vi "CommunicationTool-Ver1.vi"(0 "VISA资源名称":refnum<visa-resource-name>="COM29", 1 "SN":string, 2 "ModelNumber":string, 5 "通信协议名称":string, 9 "DelayTime":u32=1000, 11 "error in":errorcluster, 12 "Debug":bool) -> (3 "字符串数值":bool, 4 "响应":string="ÿÿÿÿÿÿÿÿÿÿÿÿÿÿÿÿÿÿÿÿÿÿÿÿÿÿÿ", 6 "反馈结果":bool, 10 "CMD":string, 14 "data":string, 15 "error out":errorcluster)   [LabVIEW 2013]
doc: "本范例根据用户指示，对串口执行读写操作。范例运行时可按下“写入”或“读取”按钮，以及修改“读数”。\n\n设置的串口参数必须匹配连接仪器或设备的参数。本范例中，“读数”参数可指定串口读取的字节数。如端口字节超过指定的字节数，超出部分将不会被读取。如端口字节数少于指定的字节数，将返回超时错误。\n\n本范例可扩展流控制选项以包括XON和XOFF，从而允许用户选择控制字符。同时，用户可启用或禁用中止符。部分设备需要通过终止符确定命令字符串的结束位置。部分设备将发送终止符以说明待读取数据的末端。本范例演示了缓冲区中检测到终止符时，结束“读取”操作或添加终止符至“写入”数据末端的方法。"
uses:
  <vilib>/Utility/NIReport.llb/NI_report.lvclass
  Ctl/Paractl.ctl
  GlobValue.vi
  <vilib>/Utility/error.llb/Error Cluster From Error Code.vi
  <vilib>/addons/_office/excel.llb/Excel Get Data ([str]).vi
  <vilib>/ErrorRing/Error Ring.xnode
  <vilib>/addons/_office/NI_ReportGenerationToolkit.lvlib
  <vilib>/Utility/NIReport.llb/Excel/NI_Excel.lvclass
panel:
  out "字符串 2":string
  out "日期/时间字符串":string
  out "times":dbl
  out "反馈前段":string
  out "Time(ms)":u32
  out "SerNO":string
  out "硬件版本":string
  out "CCID":string="PASS"
  out "生产日期":string
  out "字符串":string
  out "x-y":u32
  out "读取缓冲区":string
  in  "命令列表":u16(ring)=17 items=["启动自动化测试", "退出自动化测试", "进入待机模式", "进入工作模式", "查询ACC IO状态", "GPS定位查询", "查询GPS定位时间", "GPS可见星数", "上网模块自检", "上网模块信号强度", "查询上网模块GPRS状态", "WIFI模块自检", "外部Flash测试", "查询电池电压", "查询电源电压", "CHARGE_CTL置低", "CHARGE_CTL置高", "查询CHARGE_WAKE状态", "3G_PWR_CTL输出低电平", "3G_PWR_CTL输出高电平", "3G_RST输出低电平", "3G_RST输出高电平", "查询ANT1_S状态", "查询ANT0_S状态", "GPS_PWREN输出低电平", "GPS_PWREN输出高电平", "CAN通信接收", "CAN通信发送", "重启", "U_CTL输出低电平", "U_CTL输出高电平", "OBD_CTL输出低电平", "OBD_CTL输出高电平", "OBD_STB输出低电平", "OBD_STB输出高电平", "3G_EN输出低电平", "3G_EN输出高电平", "写入主机条码", "读出主机条码", "写入生产日期", "读出生产日期", "读出CCID", "写入终端ID", "读出终端ID", "写入硬件版本", "读出硬件版本", "查看TBC文件", "进入休眠模式", "写入APN1", "写入APN2", "读出APN1", "读出APN2", "写入WIFI名称", "写入WIFI密码", "WIFI模块自检", "读出WIFI名称", "读出WIFI密码", "查询4G固件版本", "查询平台登录状态", "读OPEN软件版本", "写入车辆TUID", "读出车辆TUID", "查询MCU软件版本", "写入证书编号", "读出证书编号", "写入供应商代码", "读出供应商代码", "写入零部件号", "读出零部件号", "读出WIFI MAC地址", "OPEN模块自检", "切断备电供电", "恢复备电供电", "检测备电电压", "检测B+电源电压", "查询平台登录状态", "SRS碰撞检测", "启动测试回环Speak", "启动测试回环Aux", "关闭测试回环", "E-call状态返回", "MIC_CTL输出低电平", "MIC_CTL输出高电平", "读取IMSI号"]
  out "Write":bool
  out "Read":bool
  out "ConfigPath":string="C:\\Users\\dell\\Desktop\\ExcelReport.vi"
  out "命令":string
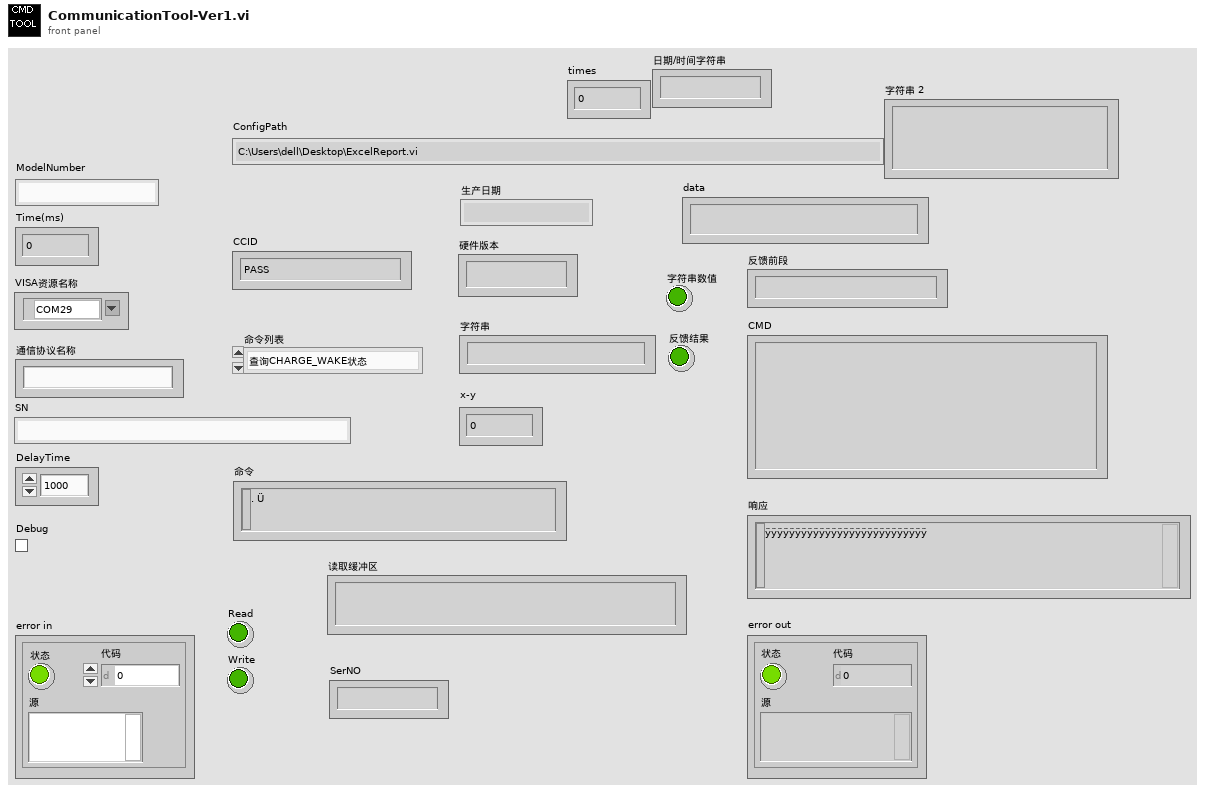
[diagram p1: front panel]
types:
  T1 = enum32{"invalid app kind", "Development System", "Run Time System", "Student Edition", "Embedded LabVIEW", "Evaluation", "Custom"}
  T2 = enum16{"maximized", "minimized", "normal", "no change"}
  T3 = enum16{"Standard Report", "HTML", "Word", "Excel"}
  T4 = typedef "Paractl.ctl" = enum16{"Fw Ver", "HW Ver", "CCID", "WiFiName", "DevID", "SN", "TUID", "CertifID", "PdTime", "Provider", "WiFiPassword", "Imei", "AuthCode", "Reserved1", "Reserved2", "Reserved3"}
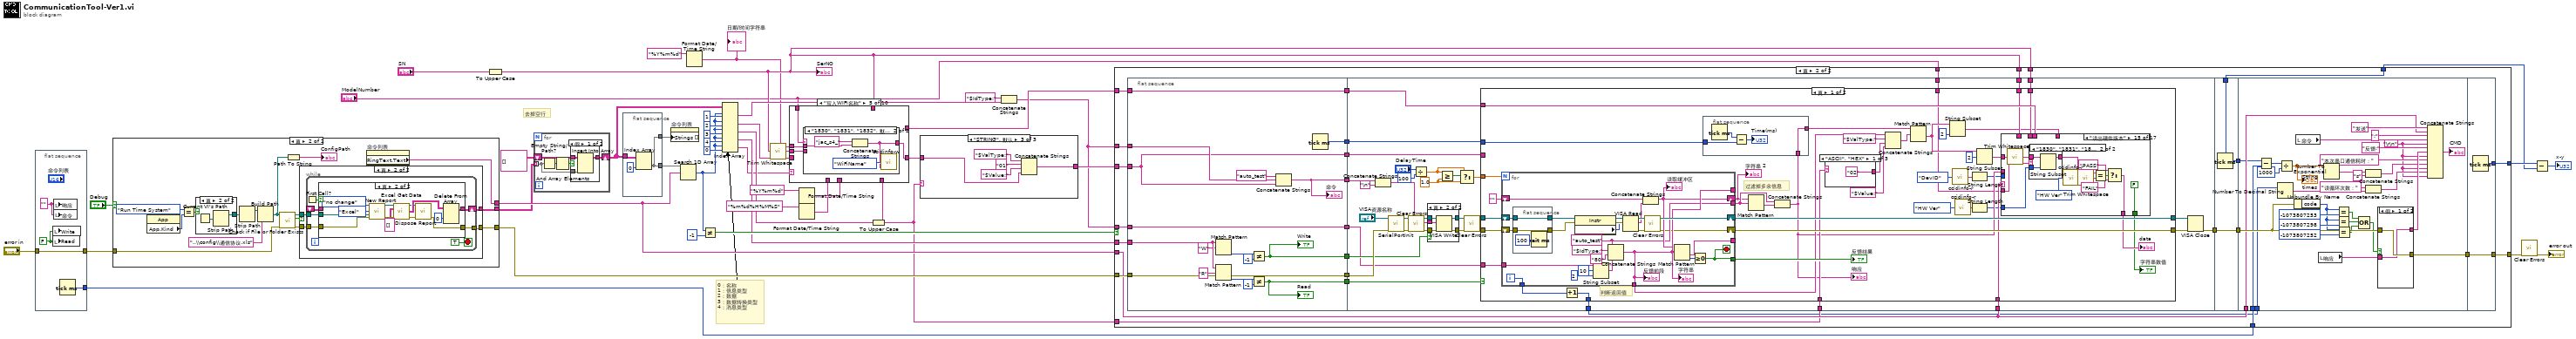
[diagram p0: block diagram]
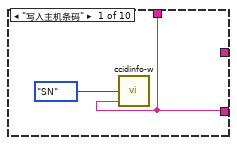
[diagram p2: hidden frame]
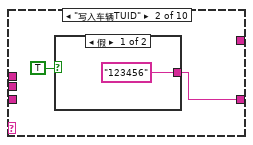
[diagram p3: hidden frame]
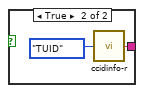
[diagram p4: hidden frame]
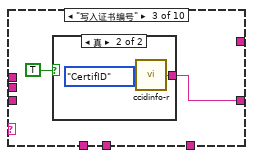
[diagram p5: hidden frame]
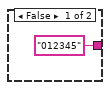
[diagram p6: hidden frame]
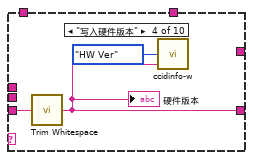
[diagram p7: hidden frame]
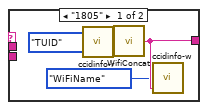
[diagram p8: hidden frame]
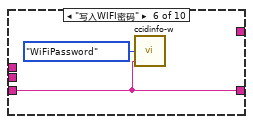
[diagram p9: hidden frame]
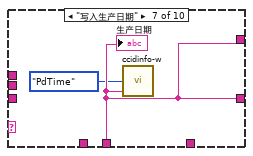
[diagram p10: hidden frame]
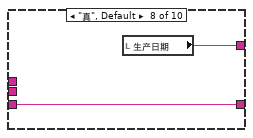
[diagram p11: hidden frame]
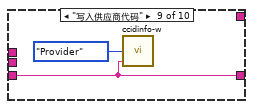
[diagram p12: hidden frame]
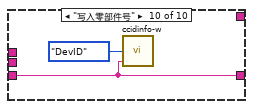
[diagram p13: hidden frame]
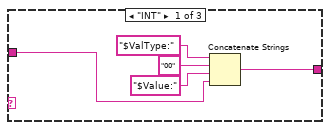
[diagram p15: hidden frame]
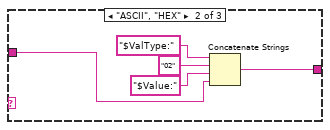
[diagram p16: hidden frame]
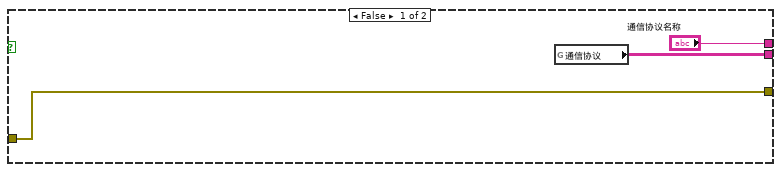
[diagram p17: hidden frame]
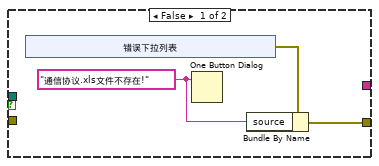
[diagram p18: hidden frame]
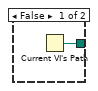
[diagram p20: hidden frame]
diagram:
  # "0：名称\n1：信息类型\n2：数据\n3：数据转换类型\n4：消息类型"
  # "去掉空行"
  n1 = flat-sequence {
    tunnel: "error in" -> [w47]
    tunnel: [w47] -> w43
    tunnel: [w46] -> w5
    frame #0 {
      w49 = FALSE ("Read")
      w48 = "" ("响应")
      n2 = local write "Write"(w49) -> ()
      n3 = local write "Read"(w49) -> ()
      n4 = local write "响应"(w48) -> ()
      n5 = local write "命令"(w48) -> ()
      n6 = Tick Count (ms)() -> (millisecond timer value=w46:u32)
    }
  }
  n7 = case shown="真" "Debug" {
    tunnel: [w51 w56] -> w41
    tunnel: w43 -> [w51 w55]
    tunnel: ["通信协议名称" w53] -> w34
    tunnel: [w50 w54] -> w19
    frame False {
      n8 = global read "GlobValue.vi" "通信协议"() -> (w50:string[][])
    }
    frame True {
      n9 = property class="App"() -> ("App.Kind"=w65:T1)  [unwired: 2 in, 2 out]
      n10 = Equal?(x=T1."Run Time System" ("y"), y=w65) -> (x = y?=w67:bool)
      n11 = case shown="真" w67 {
        tunnel: [w101 w103] -> w66
        frame False {
          n12 = Current VI's Path() -> (path=w101:path)
        }
        frame True {
          n13 = Current VI's Path() -> (path=w102:path)
          n14 = Strip Path(path=w102) -> (stripped path=w103:path)  [unwired: 1 out]
        }
      }
      n15 = Strip Path(path=w66) -> (stripped path=w60:path)  [unwired: 1 out]
      n16 = Build Path(base path=w60, name or relative path="..\\config\\通信协议.xls" ("连接的字符串")) -> (appended path=w62:path)
      n17 = call <vilib>:"Check if File or Folder Exists.vi"("error in (no error)"=w55, "path"=w62) -> ("error out"=w57:errorcluster, "file or folder exists?"=w59:bool, "dup path"=w58:path)  [unwired: 7 out]
      n18 = Path To String(path=w62) -> (string=→"ConfigPath":string)
      n19 = case shown="真" w59 {
        tunnel: w58 -> [_ w78]
        tunnel: w57 -> [_ w77]
        tunnel: [w69 w76] -> w56
        tunnel: [_ w75] -> w54
        frame False {
          w70 = "通信协议.xls文件不存在!" ("消息")
          n20 = xnode "错误下拉列表"() -> ("错误输出"=w68:errorcluster)
          n21 = One Button Dialog(message=w70) -> ()  [unwired: 1 in, 1 out]
          n22 = Bundle By Name(cluster=w68, "source"=w70) -> (w69:errorcluster)
        }
        frame True {
          n23 = while {
            tunnel: w78 -> [w84]
            tunnel: [w83] -> w76
            tunnel: w77 -> [w82]
            shift-right: [w85] -> w75
            shift-left: _ -> [w80]
            stop <- TRUE stop-if-true
            n24 = First Call?() -> (First Call?: T/F=w79:bool)
            n25 = case shown="真" w79 {
              tunnel: [w87 w91] -> w85
              tunnel: w84 -> [_ w90]
              tunnel: [w86 w89] -> w83
              tunnel: w82 -> [w86 w88]
              tunnel: w80 -> [w87 _]
              frame False {
              }
              frame True {
                n26 = call <vilib>:"New Report.vi"("window state (normal)"=T2."no change", "report type"=T3."Excel", "template (empty)"=w90, "error in (no error)"=w88) -> ("report out"=w96:refnum<class "NI_report.lvclass">, "error out"=w97:errorcluster)  [unwired: 2 in, 8 out]
                n27 = call-poly <vilib>:"Excel Get Data.vi"("report in"=w96, "data type"=string[][] [], "error in (no error)"=w97) -> ("report out"=w93:refnum<class "NI_report.lvclass">, "data"=w98:string[][], "error out"=w92:errorcluster)  [unwired: 10 in]
                n28 = call-dynamic "Dispose Report.vi"("report in"=w93, "error in (no error)"=w92) -> ("error out"=w89:errorcluster)  [unwired: 3 in, 10 out]
                n29 = Delete From Array(array=w98, index (row)=0 ("索引 (行)")) -> (array with subset deleted=w91:string[][])  [unwired: 2 in, 1 out]
              }
            }
          }
        }
      }
      n30 = property on="命令列表" class="Ring (严格)"() -> ("RingText.Text"=w53:string)  [unwired: 2 in, 2 out]
    }
  }
  n31 = To Upper Case(1:"SN") -> (0:w11:string)
  "SerNO" <- w11
  n32 = for {
    tunnel: w19 -> [w104] mode=indexing
    shift-right: [w107] -> w27
    shift-left: string[][] [] -> [w108]
    n33 = Empty String/Path?(string/path=w104) -> (empty?=w106:bool[])
    n34 = And Array Elements(Boolean array=w106) -> (logical AND=w105:bool)
    n35 = case shown="假" w105 {
      tunnel: w108 -> [w111 w112]
      tunnel: [w110 w112] -> w107
      tunnel: w104 -> [w109 _]
      frame False {
        n36 = Insert Into Array(array=w111, new element=w109) -> (w110:string[][])  [unwired: 2 in]
      }
      frame True {
      }
    }
  }
  n37 = flat-sequence {
    tunnel: [w113] -> w33
    tunnel: w27 -> [w114]
    tunnel: [w113] -> w17
    frame #0 {
      n38 = Index Array(array=w114, index (col)=0 ("禁用的索引 (列)")) -> (element=w113:string[])  [unwired: 1 in]
    }
  }
  n39 = property on="命令列表" class="Ring (严格)"("Strings []"=w17) -> ()  [unwired: 2 in, 2 out]
  n40 = Search 1D Array(1D array=w33, element=w34) -> (index of element=w16:i32)  [unwired: 1 in]
  n41 = Format Date/Time String(time format string (%c)="%Y%m%d" ("时间格式字符串(%c)")) -> (date/time string=w1:string)  [unwired: 2 in]
  "日期/时间字符串" <- w1
  n42 = Not Equal?(x=w16, y=-1) -> (x != y?=w36:bool)
  n43 = Index Array(array=w27, index (row) #1=w16, index (col) #1=1 ("索引 (列)"), index (row) #2=w16, index (col) #2=2 ("索引 (列)"), index (row) #3=w16, index (col) #3=3 ("索引 (列)"), index (row) #4=w16, index (col) #4=4 ("禁用的索引 (列)"), index (row) #5=w16, index (col) #5=0 ("禁用的索引 (列)")) -> (element #1=w13:string, element #2=w23:string, element #3=w29:string, element #4=w31:string, element #5=w15:string)
  n44 = call <vilib>:"Trim Whitespace.vi"("string"=w11) -> ("trimmed string"=w3:string)  [unwired: 1 in]
  n45 = Format Date/Time String(time format string (%c)="%Y%m%d" ("时间格式字符串(%c)")) -> (date/time string=w9:string)  [unwired: 2 in]
  n46 = Format Date/Time String(time format string (%c)="%m%d%H%M%S" ("时间格式字符串(%c)")) -> (date/time string=w7:string)  [unwired: 2 in]
  n47 = To Upper Case(1:w29) -> (0:w18:string)
  n48 = case shown="\"写入WIFI名称\"" w15 {
    tunnel: w23 -> [_ _ _ w130 _ w144 _ w148 w150 w152]
    tunnel: [w117 w119 w124 w129 w134 w144 w146 w148 w150 w152] -> w20
    tunnel: [_ _ _ _ _ _ w146 w147 _ _] -> w21
    tunnel: w11 -> [w117 _ _ _ _ _ _ _ _ _]
    tunnel: w3 -> [_ _ _ _ w132 _ _ _ _ _]
    tunnel: w18 -> [_ _ _ _ _ _ _ _ _ _]
    tunnel: w9 -> [_ _ _ _ _ _ w146 _ _ _]
    tunnel: "ModelNumber" -> [_ _ _ _ w133 _ _ _ _ _]
    tunnel: w7 -> [_ _ _ _ _ _ _ _ _ _]
    tunnel: w1 -> [_ _ _ _ w131 _ _ _ _ _]
    frame "写入主机条码" {
      n49 = call "ccidinfo-w.vi"("Data"=w117, "Data Type"=Paractl."SN") -> ()  [unwired: 2 in]
    }
    frame "写入车辆TUID" {
      n50 = case shown="假" TRUE {
        tunnel: ["123456" ("Data") w122] -> w119
        frame False {
        }
        frame True {
          n51 = call "ccidinfo-r.vi"("Data Type"=Paractl."TUID") -> ("Data"=w122:string)
        }
      }
    }
    frame "写入证书编号" {
      n52 = case shown="真" TRUE {
        tunnel: ["012345" ("Data") w127] -> w124
        frame False {
        }
        frame True {
          n53 = call "ccidinfo-r.vi"("Data Type"=Paractl."CertifID") -> ("Data"=w127:string)
        }
      }
    }
    frame "写入硬件版本" {
      n54 = call <vilib>:"Trim Whitespace.vi"("string"=w130) -> ("trimmed string"=w129:string)  [unwired: 1 in]
      "硬件版本" <- w129
      n55 = call "ccidinfo-w.vi"("Data"=w129, "Data Type"=Paractl."HW Ver") -> ()  [unwired: 2 in]
    }
    frame "写入WIFI名称" {
      n56 = case shown="\"1830\", \"1831\", \"1832\", 默认" w133 {
        tunnel: [w137 w141] -> w134
        tunnel: w132 -> [_ _]
        tunnel: w131 -> [_ w139]
        frame "1805" {
          n57 = call "ccidinfo-r.vi"("Data Type"=Paractl."TUID") -> ("Data"=w138:string)
          n58 = call "WifiConcat.vi"("TUID"=w138) -> ("WIFIName"=w137:string)
          n59 = call "ccidinfo-w.vi"("Data"=w137, "Data Type"=Paractl."WiFiName") -> ()  [unwired: 2 in]
        }
        frame "1830", "1831", "1832", Default {
          n60 = Concatenate Strings("jac_s4_" ("SerNO 2"), w139) -> (w141:string)
          n61 = call "ccidinfo-w.vi"("Data"=w141, "Data Type"=Paractl."WiFiName") -> ()  [unwired: 2 in]
        }
      }
    }
    frame "写入WIFI密码" {
      n62 = call "ccidinfo-w.vi"("Data"=w144, "Data Type"=Paractl."WiFiPassword") -> ()  [unwired: 2 in]
    }
    frame "写入生产日期" {
      n63 = call "ccidinfo-w.vi"("Data"=w146, "Data Type"=Paractl."PdTime") -> ()  [unwired: 2 in]
      "生产日期" <- w146
    }
    frame "真", Default {
      n64 = local read "生产日期"() -> (w147:string)
    }
    frame "写入供应商代码" {
      n65 = call "ccidinfo-w.vi"("Data"=w150, "Data Type"=Paractl."Provider") -> ()  [unwired: 2 in]
    }
    frame "写入零部件号" {
      n66 = call "ccidinfo-w.vi"("Data"=w152, "Data Type"=Paractl."DevID") -> ()  [unwired: 2 in]
    }
  }
  n67 = case shown="\"STRING\", 默认" w18 {
    tunnel: [w153 w158 w163] -> w35
    tunnel: w20 -> [w154 w159 w164]
    frame "INT" {
      n68 = Concatenate Strings("$ValType:", "00", "$Value:", w154) -> (w153:string)
    }
    frame "ASCII", "HEX" {
      n69 = Concatenate Strings("$ValType:", "02", "$Value:", w159) -> (w158:string)
    }
    frame "STRING", Default {
      n70 = Concatenate Strings("$ValType:", "01", "$Value:", w164) -> (w163:string)
    }
  }
  n71 = Concatenate Strings("$IdType:", w13) -> (w12:string)
  n72 = case shown="真" w36 {
    tunnel: w34 -> [w172 w191]
    tunnel: w12 -> [_ w200]
    tunnel: w35 -> [_ w199]
    tunnel: w41 -> [_ w198]
    tunnel: [w168 w196] -> w45
    tunnel: w31 -> [_ w195]
    tunnel: w18 -> [_ w177]
    tunnel: [_ w187] -> w42
    tunnel: [_ w186] -> w26
    tunnel: w21 -> [_ w185]
    tunnel: w11 -> [_ w183]
    tunnel: w11 -> [_ w182]
    tunnel: w12 -> [_ w178]
    tunnel: "ModelNumber" -> [_ w176]
    tunnel: w5 -> [_ w174]
    frame False {
      (unwired) "FF" ("响应")
      n73 = Concatenate Strings(w172, "名称不存在" ("消息")) -> (w169:string)
      n74 = One Button Dialog(message=w169) -> ()  [unwired: 1 in, 1 out]
      n75 = Bundle By Name(cluster=errorcluster {"status"=TRUE, "code"=5000, "source"=""} ("error in 1 (no error)"), "source"=w169) -> (w168:errorcluster)
    }
    frame True {
      n76 = flat-sequence {
        tunnel: w200 -> [w206]
        tunnel: w199 -> [w204]
        tunnel: w198 -> [w217]
        tunnel: [w217] -> w197
        tunnel: w195 -> [w216]
        tunnel: [w209] -> w194
        tunnel: [w208] -> w193
        tunnel: [w207] -> w192
        tunnel: w185 -> [w205]
        tunnel: [w205] -> w184
        tunnel: [w204] -> w181
        tunnel: [w203] -> w180
        tunnel: [w201] -> w179
        tunnel: w178 -> [w201]
        tunnel: w197 -> [w247]
        tunnel: w194 -> [w242]
        tunnel: w193 -> [w245]
        tunnel: [w246] -> w190
        tunnel: w192 -> [w226]
        tunnel: w191 -> [w233]
        tunnel: w184 -> [w232]
        tunnel: w183 -> [w231]
        tunnel: w182 -> [w230]
        tunnel: w181 -> [w229]
        tunnel: w180 -> [w228]
        tunnel: w179 -> [w223]
        tunnel: w177 -> [w222]
        tunnel: w176 -> [w221]
        tunnel: [w220] -> w173
        tunnel: w190 -> [w486]
        tunnel: [w486] -> w189
        tunnel: [w485] -> w186
        tunnel: [w485] -> w175
        tunnel: w189 -> [w512]
        tunnel: w191 -> [w506]
        tunnel: [w513] -> w188
        tunnel: w175 -> [w500]
        tunnel: w174 -> [w499]
        tunnel: w173 -> [w492]
        tunnel: [w524] -> w196
        tunnel: w188 -> [w524]
        tunnel: [w523] -> w187
        frame #0 {
          n77 = Match Pattern(string=w216, regular expression="W" ("正则表达式")) -> (offset past match=w210:i32)  [unwired: 1 in, 3 out]
          n78 = Match Pattern(string=w216, regular expression="R" ("正则表达式")) -> (offset past match=w211:i32)  [unwired: 1 in, 3 out]
          n79 = Not Equal?(x=w210, y=-1) -> (x != y?=w209:bool)
          "Write" <- w209
          n80 = Not Equal?(x=w211, y=-1) -> (x != y?=w208:bool)
          "Read" <- w208
          n81 = Concatenate Strings("auto_test", w206, w204) -> (w207:string)
          "命令" <- w207
          n82 = Tick Count (ms)() -> (millisecond timer value=w203:u32)
        }
        frame #1 {
          w239 = 1.0 ("y")
          n83 = Concatenate Strings(w226, "\n") -> (w224:string)
          n84 = call "SerialPortInit.vi"("错误输入"=w247, "COMIn"="VISA资源名称") -> ("错误输出"=w243:errorcluster, "COMOut"=w244:refnum<visa-resource-name>)  [unwired: 8 in]
          n85 = call <vilib>:"Clear Errors.vi"("error in (no error)"=w243) -> ("error out"=w219:errorcluster)  [unwired: 6 in]
          n86 = Divide(x="DelayTime", y=u32 100) -> (x/y=w238:dbl)
          n87 = case shown="真" w242 {
            tunnel: w244 -> [w251 w256]
            tunnel: [w251 w255] -> w241
            tunnel: [w250 w254] -> w240
            tunnel: w219 -> [w250 w253]
            tunnel: w224 -> [_ w252]
            frame False {
            }
            frame True {
              n88 = VISA Write(VISA resource name=w256, write buffer=w252, error in (no error)=w253) -> (VISA resource name out=w255:refnum<visa-resource-name>, error out=w254:errorcluster)  [unwired: 1 out]
            }
          }
          n89 = Greater Or Equal?(x=w238, y=w239) -> (x >= y?=w237:bool)
          n90 = Select(t=w238, s=w237, f=w239) -> (s? t:f=w234:dbl)
          n91 = call <vilib>:"Clear Errors.vi"("error in (no error)"=w240) -> ("error out"=w218:errorcluster)  [unwired: 6 in]
          n92 = case shown="真" w245 {
            tunnel: [w295 w484] -> w248
            tunnel: w241 -> [w294 w484]
            tunnel: [w296 w483] -> w249
            tunnel: w218 -> [w293 w483]
            tunnel: w234 -> [w291 _]
            tunnel: w233 -> [w290 _]
            tunnel: w232 -> [w287 _]
            tunnel: w231 -> [w286 _]
            tunnel: w230 -> [w285 _]
            tunnel: w229 -> [_ _]
            tunnel: w228 -> [w284 _]
            tunnel: w223 -> [w281 _]
            tunnel: w222 -> [w280 _]
            tunnel: w221 -> [w266 _]
            tunnel: [w264 _] -> w220
            frame True {
              # "过滤掉多余信息"
              # "判断返回值"
              n93 = for {
                N: w291 -> [_]
                shift-right: [w455] -> w296
                shift-left: w293 -> [w470]
                shift-right: [w458] -> w257
                shift-left: "" ("read buffer") -> [w474]
                shift-right: [w478] -> w295
                shift-left: w294 -> [w469]
                tunnel: [w468] -> w282
                tunnel: [w459] -> _
                tunnel: w281 -> [w466]
                tunnel: [w460] -> _
                tunnel: [w459] -> w279
                tunnel: [w457] -> w269
                tunnel: [w456] -> w265
                i -> [w456]
                stop <- w468 stop-if-true
                w457 = "auto_test"
                n94 = flat-sequence {
                  tunnel: w470 -> [w482]
                  tunnel: [w482] -> w471
                  tunnel: [w481] -> w472
                  tunnel: w469 -> [w481]
                  frame #0 {
                    n95 = Wait (ms)(milliseconds to wait=u32 100 ("等待时间（毫秒）")) -> ()  [unwired: 1 out]
                  }
                }
                n96 = property class="Instr"(reference=w472, error in=w471) -> (reference out=w477:refnum<visa-resource-name>, error out=w476:errorcluster, "Serial Settings:Number of Bytes at Serial Port"=w475:u32)
                n97 = String Subset(string=w466, offset (0)=10 ("偏移量(0)"), length (rest)=2 ("长度（剩余）")) -> (substring=w467:string)
                n98 = Concatenate Strings(w457, "$IdType:", "80" ("字符串"), w467) -> (w459:string)
                "字符串" <- w459
                "反馈前段" <- w459
                n99 = VISA Read(VISA resource name=w477, byte count=w475, error in (no error)=w476) -> (VISA resource name out=w478:refnum<visa-resource-name>, read buffer=w473:string, error out=w479:errorcluster)  [unwired: 1 out]
                n100 = Concatenate Strings(w474, w473) -> (w458:string)
                "读取缓冲区" <- w458
                n101 = call <vilib>:"Clear Errors.vi"("error in (no error)"=w479) -> ("error out"=w455:errorcluster)  [unwired: 6 in]
                n102 = Match Pattern(string=w458, regular expression=w459) -> (after substring=w460:string, offset past match=w461:i32)  [unwired: 1 in, 2 out]
                n103 = Greater Or Equal To 0?(x=w461) -> (x >= 0?=w468:bool)
              }
              "反馈结果" <- w282
              "字符串 2" <- w257
              n104 = Increment(x=w265) -> (x+1=w264:i32)
              n105 = flat-sequence {
                tunnel: w284 -> [w452]
                tunnel: w267 -> [w451]
                tunnel: [w451] -> w283
                frame #0 {
                  n106 = Tick Count (ms)() -> (millisecond timer value=w453:u32)
                  n107 = Subtract(x=w453, y=w452) -> (x-y=→"Time(ms)":u32)
                }
              }
              n108 = Match Pattern(string=w257, regular expression=w269) -> (after substring=w268:string)  [unwired: 1 in, 3 out]
              n109 = Concatenate Strings(w269, w268) -> (w267:string)
              "响应" <- w267
              n110 = case shown="\"ASCII\", \"HEX\"" w280 {
                tunnel: ["02" "01" "00"] -> w277
                frame "ASCII", "HEX" {
                }
                frame "STRING", Default {
                }
                frame "INT" {
                }
              }
              n111 = Concatenate Strings(w279, "$ValType:", w277, "$Value:") -> (w275:string)
              n112 = Match Pattern(string=w283, regular expression=w275) -> (after substring=w270:string)  [unwired: 1 in, 3 out]
              n113 = String Subset(string=w270, length (rest)=2) -> (substring=w273:string)  [unwired: 1 in]
              n114 = call "ccidinfo-r.vi"("Data Type"=Paractl."DevID") -> ("Data"=w262:string)
              n115 = call "ccidinfo-r.vi"("Data Type"=Paractl."HW Ver") -> ("Data"=w259:string)
              n116 = String Length(string=w262) -> (length=w261:i32)
              n117 = String Length(string=w259) -> (length=w258:i32)
              n118 = String Subset(string=w270, offset (0)=2) -> (substring=w271:string)  [unwired: 1 in]
              n119 = case shown="\"读出硬件版本\"" w290 {
                tunnel: [w301 w305 w311 w318 w327 w336 w345 w357 w372 w379 w388 w402 w410 w416 w427 w437 w449] -> w289
                tunnel: [FALSE FALSE TRUE FALSE FALSE FALSE FALSE FALSE FALSE FALSE FALSE FALSE FALSE FALSE FALSE TRUE TRUE] -> w288
                tunnel: w273 -> [w302 _ _ _ _ _ _ _ _ _ _ w398 _ _ _ _ _]
                tunnel: w287 -> [_ _ _ _ _ _ _ _ _ _ _ _ _ _ _ _ _]
                tunnel: w286 -> [_ _ _ _ _ _ _ _ _ _ _ _ _ _ _ _ _]
                tunnel: w285 -> [_ _ _ _ _ _ _ _ _ _ _ _ _ _ _ _ _]
                tunnel: w267 -> [_ _ _ _ _ _ _ _ _ _ _ _ _ _ _ _ _]
                tunnel: w271 -> [_ w306 w310 w317 w326 w335 w344 w356 w369 w378 w386 w400 w409 w417 w426 w439 w450]
                tunnel: w266 -> [_ _ _ _ _ _ _ w352 _ _ _ _ _ _ w420 w436 _]
                tunnel: w261 -> [_ _ _ _ _ _ _ w351 _ _ _ _ _ _ _ _ _]
                tunnel: w258 -> [_ _ _ _ _ _ _ _ _ _ _ _ _ _ w419 _ _]
                frame "真", Default {
                  n120 = Empty String/Path?(string/path=w302) -> (empty?=w303:bool)
                  n121 = Select(t="", s=w303, f=w302) -> (s? t:f=w301:string)
                }
                frame "E-call状态返回", "查询4G固件版本", "读OPEN软件版本" {
                  n122 = call <vilib>:"Trim Whitespace.vi"("string"=w306) -> ("trimmed string"=w305:string)  [unwired: 1 in]
                }
                frame "读出WIFI MAC地址" {
                  n123 = call <vilib>:"Trim Whitespace.vi"("string"=w310) -> ("trimmed string"=w309:string)  [unwired: 1 in]
                  n124 = String Length(string=w309) -> (length=w312:i32)
                  n125 = call "ccidinfo-w.vi"("Data"=w309, "Data Type"=Paractl."Reserved3") -> ()  [unwired: 2 in]
                  n126 = Number To Decimal String(number=w312) -> (decimal integer string=w311:string)  [unwired: 1 in]
                }
                frame "读出主机条码" {
                  n127 = call <vilib>:"Trim Whitespace.vi"("string"=w317) -> ("trimmed string"=w314:string)  [unwired: 1 in]
                  n128 = call "ccidinfo-r.vi"("Data Type"=Paractl."SN") -> ("Data"=w315:string)
                  n129 = Equal?(x=w314, y=w315) -> (x = y?=w321:bool)
                  n130 = Select(t="PASS" ("string"), s=w321, f="FAIL") -> (s? t:f=w318:string)
                }
                frame "读出车辆TUID" {
                  n131 = call <vilib>:"Trim Whitespace.vi"("string"=w326) -> ("trimmed string"=w324:string)  [unwired: 1 in]
                  n132 = call "ccidinfo-r.vi"("Data Type"=Paractl."TUID") -> ("Data"=w325:string)
                  n133 = Equal?(x=w324, y=w325) -> (x = y?=w330:bool)
                  n134 = Select(t="PASS" ("string"), s=w330, f="FAIL") -> (s? t:f=w327:string)
                }
                frame "读出证书编号" {
                  n135 = call <vilib>:"Trim Whitespace.vi"("string"=w335) -> ("trimmed string"=w333:string)  [unwired: 1 in]
                  n136 = call "ccidinfo-r.vi"("Data Type"=Paractl."CertifID") -> ("Data"=w334:string)
                  n137 = Equal?(x=w333, y=w334) -> (x = y?=w339:bool)
                  n138 = Select(t="PASS" ("string"), s=w339, f="FAIL") -> (s? t:f=w336:string)
                }
                frame "读出供应商代码" {
                  n139 = call <vilib>:"Trim Whitespace.vi"("string"=w344) -> ("trimmed string"=w342:string)  [unwired: 1 in]
                  n140 = call "ccidinfo-r.vi"("Data Type"=Paractl."Provider") -> ("Data"=w343:string)
                  n141 = Equal?(x=w342, y=w343) -> (x = y?=w348:bool)
                  n142 = Select(t="PASS" ("string"), s=w348, f="FAIL") -> (s? t:f=w345:string)
                }
                frame "读出零部件号" {
                  n143 = call <vilib>:"Trim Whitespace.vi"("string"=w356) -> ("trimmed string"=w354:string)  [unwired: 1 in]
                  n144 = case shown="\"1805\"" w352 {
                    tunnel: w354 -> [w362 w365]
                    tunnel: [w362 w364] -> w353
                    tunnel: w351 -> [_ w363]
                    frame "1805" {
                    }
                    frame "1830", "1831", "1832", Default {
                      n145 = String Subset(string=w365, length (rest)=w363) -> (substring=w364:string)  [unwired: 1 in]
                    }
                  }
                  n146 = call "ccidinfo-r.vi"("Data Type"=Paractl."DevID") -> ("Data"=w355:string)
                  n147 = Equal?(x=w353, y=w355) -> (x = y?=w360:bool)
                  n148 = Select(t="PASS" ("string"), s=w360, f="FAIL") -> (s? t:f=w357:string)
                }
                frame "读出WIFI名称" {
                  n149 = call <vilib>:"Trim Whitespace.vi"("string"=w369) -> ("trimmed string"=w367:string)  [unwired: 1 in]
                  n150 = call "ccidinfo-r.vi"("Data Type"=Paractl."WiFiName") -> ("Data"=w370:string)
                  n151 = Equal?(x=w367, y=w370) -> (x = y?=w371:bool)
                  n152 = Select(t="PASS" ("string"), s=w371, f="FAIL") -> (s? t:f=w372:string)
                }
                frame "读出WIFI密码" {
                  w375 = Paractl."WiFiPassword" ("Data Type")
                  n153 = call <vilib>:"Trim Whitespace.vi"("string"=w378) -> ("trimmed string"=w377:string)  [unwired: 1 in]
                  n154 = call "ccidinfo-r.vi"("Data Type"=w375) -> ("Data"=w376:string)
                  n155 = call "ccidinfo-w.vi"("Data"=w377, "Data Type"=w375) -> ()  [unwired: 2 in]
                  n156 = Equal?(x=w377, y=w376) -> (x = y?=w382:bool)
                  n157 = Select(t="PASS" ("string"), s=w382, f="FAIL") -> (s? t:f=w379:string)
                }
                frame "读出CCID" {
                  n158 = call <vilib>:"Trim Whitespace.vi"("string"=w386) -> ("trimmed string"=w385:string)  [unwired: 1 in]
                  n159 = String Length(string=w385) -> (length=w391:i32)
                  n160 = Equal?(x=w391, y=20) -> (x = y?=w389:bool)
                  n161 = To Upper Case(1:w385) -> (0:w387:string)
                  "CCID" <- w387
                  n162 = Select(t="PASS" ("string"), s=w389, f="FAIL") -> (s? t:f=w388:string)
                  n163 = call "ccidinfo-w.vi"("Data"=w387, "Data Type"=Paractl."CCID") -> ()  [unwired: 2 in]
                }
                frame "读取IMSI号" {
                  n164 = call <vilib>:"Trim Whitespace.vi"("string"=w400) -> ("trimmed string"=w399:string)  [unwired: 1 in]
                  n165 = Equal?(x=w398, y="01") -> (x = y?=w396:bool)
                  n166 = To Upper Case(1:w399) -> (0:w401:string)
                  n167 = Select(t="PASS" ("string"), s=w396, f="FAIL") -> (s? t:f=w402:string)
                  n168 = call "ccidinfo-w.vi"("Data"=w401, "Data Type"=Paractl."Imei") -> ()  [unwired: 2 in]
                }
                frame "读出生产日期" {
                  n169 = call <vilib>:"Trim Whitespace.vi"("string"=w409) -> ("trimmed string"=w407:string)  [unwired: 1 in]
                  n170 = call "ccidinfo-r.vi"("Data Type"=Paractl."PdTime") -> ("Data"=w408:string)
                  n171 = Equal?(x=w407, y=w408) -> (x = y?=w413:bool)
                  n172 = Select(t="PASS" ("string"), s=w413, f="FAIL") -> (s? t:f=w410:string)
                }
                frame "查询MCU软件版本" {
                  n173 = call <vilib>:"Trim Whitespace.vi"("string"=w417) -> ("trimmed string"=w416:string)  [unwired: 1 in]
                  n174 = call "ccidinfo-w.vi"("Data"=w416, "Data Type"=Paractl."HW Ver") -> ()  [unwired: 2 in]
                }
                frame "读出硬件版本" {
                  n175 = call <vilib>:"Trim Whitespace.vi"("string"=w426) -> ("trimmed string"=w423:string)  [unwired: 1 in]
                  n176 = case shown="\"1830\", \"1831\", \"1832\", 默认" w420 {
                    tunnel: w423 -> [w432 w435]
                    tunnel: [w432 w434] -> w421
                    tunnel: w419 -> [_ w433]
                    frame "1805" {
                    }
                    frame "1830", "1831", "1832", Default {
                      n177 = String Subset(string=w435, length (rest)=w433) -> (substring=w434:string)  [unwired: 1 in]
                    }
                  }
                  n178 = call "ccidinfo-r.vi"("Data Type"=Paractl."HW Ver") -> ("Data"=w424:string)
                  n179 = call <vilib>:"Trim Whitespace.vi"("string"=w424) -> ("trimmed string"=w422:string)  [unwired: 1 in]
                  n180 = Equal?(x=w421, y=w422) -> (x = y?=w430:bool)
                  n181 = Select(t="PASS" ("string"), s=w430, f="FAIL") -> (s? t:f=w427:string)
                }
                frame "检测B+电源电压", "检测备电电压" {
                  n182 = case shown="\"1805\"" w436 {
                    tunnel: w439 -> [w446 w447]
                    tunnel: [w441 w447] -> w437
                    frame "1805" {
                      n183 = call <vilib>:"Trim Whitespace.vi"("string"=w446) -> ("trimmed string"=w445:string)  [unwired: 1 in]
                      n184 = String To Byte Array(string=w445) -> (unsigned byte array=w444:u8[])
                      n185 = Index Array(array=w444) -> (element=w442:u8)  [unwired: 1 in]
                      n186 = Divide(x=w442, y=10) -> (x/y=w440:dbl)
                      n187 = Number To Fractional String(number=w440) -> (F-format string=w441:string)  [unwired: 3 in]
                    }
                    frame "1830", "1831", "1832", Default {
                    }
                  }
                }
                frame "上网模块信号强度" {
                  n188 = call <vilib>:"Trim Whitespace.vi"("string"=w450) -> ("trimmed string"=w449:string)  [unwired: 1 in]
                }
              }
              "data" <- w289
              "字符串数值" <- w288
            }
            frame False {
            }
          }
          n189 = VISA Close(VISA resource name=w248, error in (no error)=w249) -> (error out=w246:errorcluster)
        }
        frame #2 {
          n190 = Tick Count (ms)() -> (millisecond timer value=w485:u32)
        }
        frame #3 {
          w487 = "\r\n"
          n191 = Subtract(x=w500, y=w499) -> (x-y=w498:u32)
          n192 = Number To Decimal String(number=w492) -> (decimal integer string=w489:string)  [unwired: 1 in]
          n193 = Divide(x=w498, y=1000) -> (x/y=w496:dbl)
          "times" <- w496
          n194 = Unbundle By Name(w512) -> ("code"=w509:i32)
          n195 = local read "命令"() -> (w501:string)
          n196 = local read "响应"() -> (w507:string)
          n197 = Number To Exponential String(number=w496) -> (E-format string=w494:string)  [unwired: 3 in]
          n198 = Equal?(x=w509, y=-1073807253) -> (x = y?=w505:bool)
          n199 = Equal?(x=w509, y=-1073807298) -> (x = y?=w504:bool)
          n200 = Equal?(x=w509, y=-1073807252) -> (x = y?=w503:bool)
          n201 = Compound Arithmetic op=OR(w505, w504, w503) -> (w502:bool)
          n202 = Concatenate Strings(w494, "s") -> (w493:string)
          n203 = Concatenate Strings("读循环次数：" ("字符串"), w489) -> (w488:string)
          n204 = case shown="假" w502 {
            tunnel: [w520 errorcluster {"status"=FALSE, "code"=0, "source"=""} ("t")] -> w513
            tunnel: w512 -> [w520 _]
            tunnel: w507 -> [w519 _]
            tunnel: [w519 ""] -> w511
            frame False {
            }
            frame True {
            }
          }
          n205 = Concatenate Strings("发送" ("字符串"), w506, ":" ("字符串"), w501, w487, "反馈:" ("字符串"), w511, w487, "本次串口通信耗时：", w493, w487, w488, w487) -> (→"CMD":string)
        }
        frame #4 {
          n206 = Tick Count (ms)() -> (millisecond timer value=w523:u32)
        }
      }
    }
  }
  n207 = call <vilib>:"Clear Errors.vi"("error in (no error)"=w45) -> ("error out"=→"error out":errorcluster)  [unwired: 6 in]
  n208 = Subtract(x=w42, y=w26) -> (x-y=→"x-y":u32)
